vi "PDDA Partial Density of Dry in Humid Air (Kg to m^3).vi"(1 "Total Pressure of Humid Air":dbl[unit], 2 "Tceg":dbl[unit], 3 "RH":dbl) -> (0 "PDDA":dbl[unit])   [LabVIEW 2018]
panel:
  out "R 2":dbl[unit]
  out "R":dbl[unit]
  out "PDDA\nPartial Density of Dry \nin Humid Air\nPDDA=(PPDA*M_da)/(R*Tk)":dbl[unit](knob) scale=0.3..1.0
  out "Temprature Of Input Air\nKelvin Degree":dbl[unit](slide) scale=273.0..373.0
  out "Tk":dbl[unit]
  out "Temprature Of Input Air\nCentigrade Degree":dbl[unit](slide) scale=0.0..100.0
  out "Humidity of Input Air":dbl(knob) scale=0.0..100.0
  out "M-da 2":dbl[unit]=0.029
  out "M-da":dbl[unit]=0.029
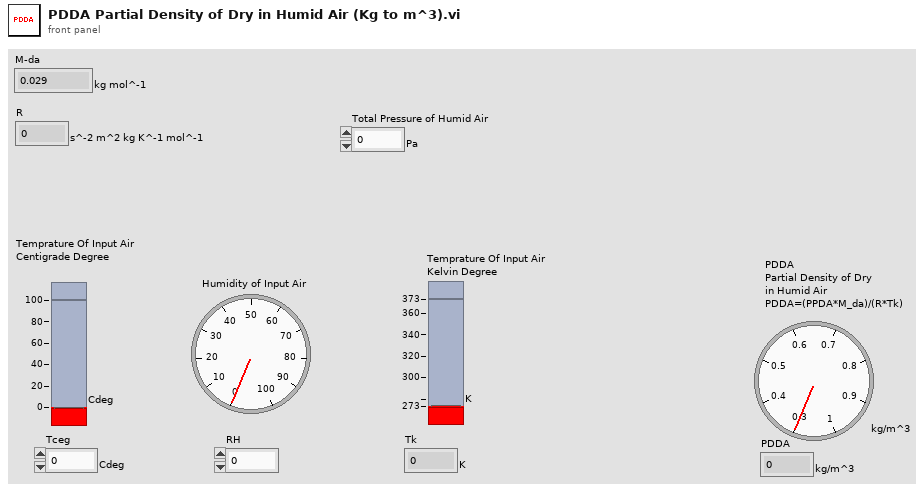
[diagram p1: front panel]
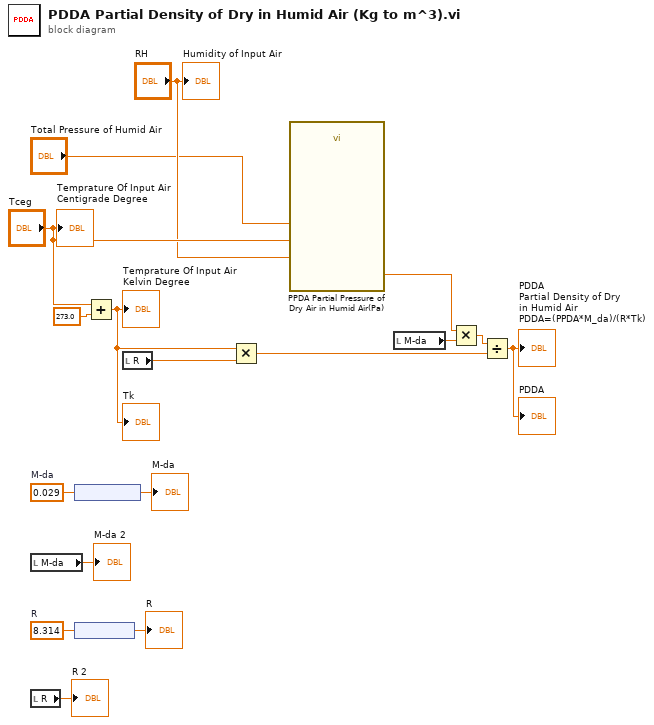
[diagram p0: block diagram]
diagram:
  w10 = 8.314  # R
  w16 = 0.029  # M-da
  n1 = local read "M-da"() -> (→"M-da 2":dbl[unit])
  n2 = local read "R"() -> (→"R 2":dbl[unit])
  n3 = node(w16) -> (→"M-da":dbl[unit])
  n4 = node(w10) -> (→"R":dbl[unit])
  n5 = Add(x="Tceg", y=dbl[unit] 273.0) -> (x+y=w6:dbl[unit])
  "Tk" <- w6
  "Temprature Of Input Air\nKelvin Degree" <- w6
  n6 = local read "R"() -> (w7:dbl[unit])
  n7 = Multiply(x=w6, y=w7) -> (x*y=w12:dbl[unit])
  n8 = call "PPDA Partial Pressure of Dry Air in Humid Air(Pa).vi"("Total Pressure of Humid Air"="Total Pressure of Humid Air", "Tceg"="Tceg", "RH"="RH") -> ("PPDA"=w2:dbl[unit])
  n9 = local read "M-da"() -> (w3:dbl[unit])
  n10 = Multiply(x=w2, y=w3) -> (x*y=w13:dbl[unit])
  n11 = Divide(x=w13, y=w12) -> (x/y=→"PDDA\nPartial Density of Dry \nin Humid Air\nPDDA=(PPDA*M_da)/(R*Tk)" →"PDDA":dbl[unit])
  "Humidity of Input Air" <- "RH"
  "Temprature Of Input Air\nCentigrade Degree" <- "Tceg"
